vi "Add App Build.vi"(6 "Project Path (Autodetect)":path, 7 "App Build (Default)":refnum<class "Build.lvclass">, 8 "error in (no error)":errorcluster, 9 "Build Spec":string, 10 "Target":string, 11 "Builder in":refnum<class "Builder.lvclass">) -> (0 "error out":errorcluster, 3 "Builder out":refnum<class "Builder.lvclass">)   [LabVIEW 2020, in "Builder Tools.lvlib" / "Builder.lvclass"]
uses:
  Builder.lvclass
  Builder.lvclass/Builder.ctl
  Build/Build.lvclass
  App Build/App Build.lvclass
  Build Info.ctl
  Builder Tools.lvlib
  Build Step.ctl
  C:/dev/lv20CE/relink/lv-builder/Builder Tools/App Build/App Build.lvclass
  C:/dev/lv20CE/relink/lv-builder/Builder Tools/Build/Build.lvclass
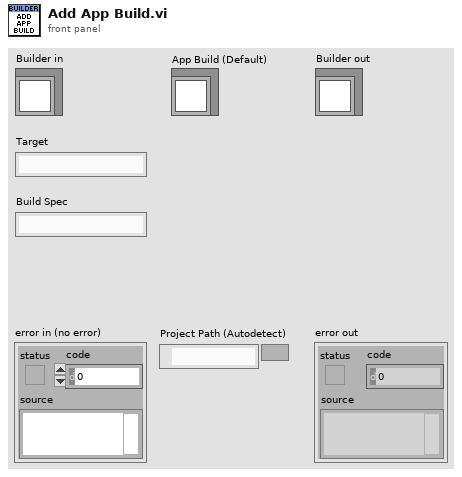
[diagram p1: front panel]
types:
  T1 = typedef "Builder Tools.lvlib/Build Info.ctl" = cluster{"Project Path":path, "Target":string, "Build Spec":string}
  T2 = typedef "Builder Tools.lvlib/Builder.lvclass/Build Step.ctl" = cluster{"Info":T1, "Build":refnum<class "Build.lvclass">}
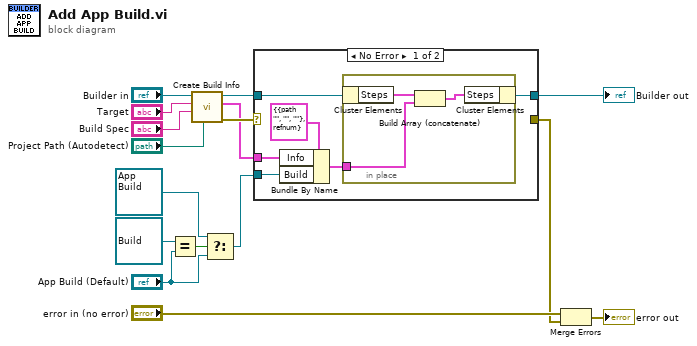
[diagram p0: block diagram]
diagram:
  n1 = Equal?(x=refnum<class "Build.lvclass"> refnum, y="App Build (Default)") -> (x = y?=w13:bool)
  n2 = call "Create Build Info.vi"("Project Path (Autodetect)"="Project Path (Autodetect)", "Build Spec"="Build Spec", "Target"="Target", "Builder in"="Builder in") -> ("error out"=w16:errorcluster, "Build Info"=w6:T1, "Builder out"=w7:refnum<class "Builder.lvclass">)  [unwired: 5 in]
  n3 = Select(t=refnum<class "App Build.lvclass"> refnum ("Builder Tools.lvlib:App Build.lvclass"), s=w13, f="App Build (Default)") -> (s? t:f=w10:refnum<class "Build.lvclass">)
  n4 = case shown="No Error" w16 {
    selector: w16 -> [_ w26]
    tunnel: w10 -> [w21 _]
    tunnel: [w19 w27] -> w8
    tunnel: w7 -> [w18 w27]
    tunnel: w6 -> [w17 _]
    tunnel: [_ w26] -> w1
    frame No Error {
      n5 = Bundle By Name(cluster=T2 {"Info"={"Project Path"=path "", "Target"="", "Build Spec"=""}, "Build"=refnum} ("Build Step"), "Info"=w17, "Build"=w21) -> (w20:T2)
      n6 = in-place {
        in-place-border: w20 -> [w24]
        n7 = in-place-cluster #1(w18) -> ("Steps"=w25:T2[])
        n8 = Build Array (concatenate)(w25, w24) -> (w23:T2[])
        n9 = in-place-cluster #1("Steps"=w23) -> (w19:refnum<class "Builder.lvclass">)
      }
    }
    frame Error {
    }
  }
  "Builder out" <- w8
  n10 = Merge Errors("error in (no error)", w1) -> (→"error out":errorcluster)
